vi "Frame History Process.vi"(8 "error in (no error)":errorcluster, 11 "Video Processor in":refnum<class "Video Cam Processor.lvclass">) -> (0 "error out":errorcluster, 2 "Depth Values Out":dbl[](array[numeric]), 3 "Video Processor out":refnum<class "Video Cam Processor.lvclass">)   [LabVIEW 2018, in "Video Cam Processor.lvclass"]
uses:
  Video Cam Processor.lvclass
  C:/Users/aaron.jencks/Documents/GitHub/emerson_seed_object_detection/LabVIEW/Projects/Paul's Video Viewer/Classes/Video File/Video File.lvclass
  Video Cam Processor.lvclass/Video Cam Processor.ctl
  ROIed Video Frame/ROIed Video Frame.lvclass
  71e46689-bb2a-4b9a-8bce-a8b402d929f4.vi
  5f884b59-f88d-4658-ba46-cdc5c40801d7.vi
  9a806c0a-74ab-44c4-a45d-9acd662e7846.vi
  5077b436-ed02-4adf-871d-4bba1f484b5e.vi
  <vilib>/Analysis/baseanly.llb/Mean (DBL).vi
  9a806c0a-74ab-44c4-a45d-9acd662e7846.vi/bd407ed1-f3fe-4715-b133-6b7bee2ad5b9.vi
  <vilib>/Analysis/NI_AALBase.lvlib
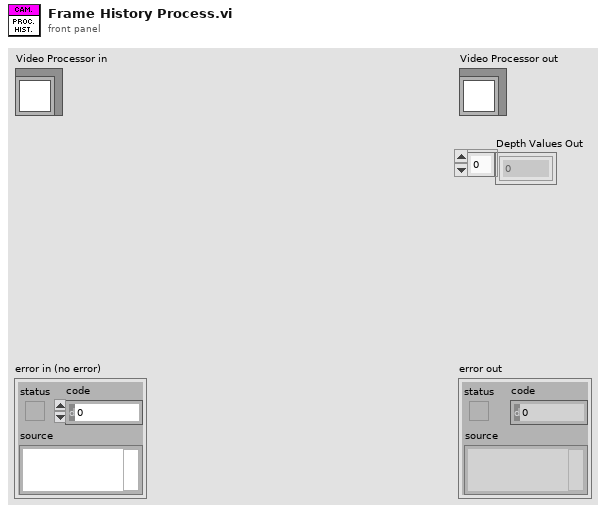
[diagram p1: front panel]
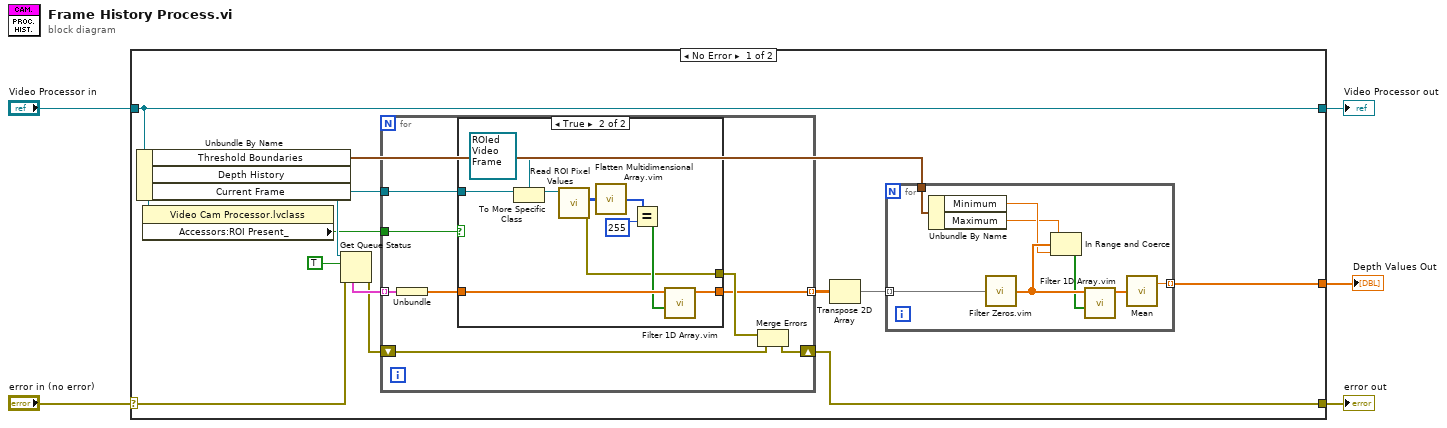
[diagram p0: block diagram]
diagram:
  n1 = case shown="No Error" "error in (no error)" {
    selector: "error in (no error)" -> [w10 w47]
    tunnel: [w12 w47] -> w4
    tunnel: [w14 w46] -> w2
    tunnel: "Video Processor in" -> [w14 w46]
    tunnel: [w6 _] -> w1
    frame No Error {
      n2 = Unbundle By Name(w14) -> ("Threshold Boundaries"=w7:cluster{"Minimum":dbl, "Maximum":dbl}, "Depth History"=w18:refnum<queue>, "Current Frame"=w15:refnum<class "Video Frame.lvclass">)
      n3 = property class="Video Cam Processor.lvclass"(reference=w14) -> ("Accessors:ROI Present_"=w13:bool)  [unwired: 1 in, 2 out]
      n4 = Get Queue Status(queue=w18, return elements? (F)=TRUE, error in (no error)=w10) -> (error out=w11:errorcluster, elements=w16:cluster{"Array":dbl[]}[])  [unwired: 6 out]
      n5 = for {
        tunnel: w16 -> [w34] mode=indexing
        tunnel: w15 -> [w33]
        tunnel: [w27] -> w9 mode=indexing
        tunnel: w13 -> [w31]
        shift-right: [w30] -> w12
        shift-left: w11 -> [w29]
        n6 = Unbundle(w34) -> ("Array"=w32:dbl[])
        n7 = case shown="True" w31 {
          tunnel: w33 -> [_ w38]
          tunnel: w32 -> [w35 w42]
          tunnel: [w35 w40] -> w27
          tunnel: [_ w36] -> w28
          frame False {
          }
          frame True {
            n8 = To More Specific Class(target class=refnum<class "ROIed Video Frame.lvclass"> refnum ("ROIed Video Frame.lvclass"), reference=w38) -> (specific class reference=w39:refnum<class "ROIed Video Frame.lvclass">)  [unwired: 1 in, 1 out]
            n9 = call-dynamic "Read ROI Pixel Values.vi"("ROIed Video Frame in"=w39) -> ("error out"=w36:errorcluster, "ROI Pixel Values"=w45:u8[][])  [unwired: 8 in, 1 out]
            n10 = call "Flatten Multidimensional Array.vim"("Array"=w45) -> ("output array"=w44:u8[])  [unwired: 14 in]
            n11 = Equal?(x=w44, y=u8 255) -> (x = y?=w41:bool[])
            n12 = call "Filter 1D Array.vim"("Boolean Filter"=w41, "Array"=w42) -> ("Array Out"=w40:dbl[])  [unwired: 9 in]
          }
        }
        n13 = Merge Errors(w28, w29) -> (w30:errorcluster)
      }
      n14 = Transpose 2D Array(2D array=w9) -> (transposed array=w8:dbl[][])
      n15 = for {
        tunnel: w8 -> [w21] mode=indexing
        tunnel: w7 -> [w22]
        tunnel: [w20] -> w6 mode=indexing
        n16 = Unbundle By Name(w22) -> ("Minimum"=w25:dbl, "Maximum"=w24:dbl)
        n17 = call "Filter Zeros.vim"("Array"=w21) -> ("Array Out"=w26:dbl[])  [unwired: 14 in]
        n18 = In Range and Coerce(upper limit=w24, x=w26, lower limit=w25) -> (In Range?=w23:bool[])  [unwired: 1 out]
        n19 = call "Filter 1D Array.vim"("Boolean Filter"=w23, "Array"=w26) -> ("Array Out"=w19:dbl[])  [unwired: 9 in]
        n20 = call-poly <vilib>:"Mean.vi"("X"=w19) -> ("mean"=w20:dbl)  [unwired: 1 out]
      }
    }
    frame Error {
    }
  }
  "error out" <- w4
  "Video Processor out" <- w2
  "Depth Values Out" <- w1
